vi "Read Waveform (Multiple).vi"(8 "error in (no error)":errorcluster, 9 "Maximum Time (5000 ms)":u32=5000, 10 "Channels":u16[](array[ring])=[1, 2] items=["Channel 1"=1, "Channel 2"=2], 11 "VISA resource name":refnum<visa-resource-name>) -> (0 "error out":errorcluster, 2 "Waveform Data":dbl[][](graph), 3 "VISA resource name out":refnum<visa-resource-name>)   [LabVIEW 2015, in "ZhiYuan ZDS Series for TCP.lvlib"]
doc: "Initiates an acquisition on all channels that you enabled with the Configure Channel VI. The VI waits for the acquisition to complete and returns the waveform for the <B>Source Channel</B> you specified. If the oscilloscope did not complete the acquisition within the time period you specify with the <B>Timeout</B> control, the VI returns a timeout error. A common cause for a timeout error is the acquisition was not triggered. For example, the trigger level is out of range of the waveform. \n\n<B>Note:</B> If your instrument does not support auto compensation for probe attenuation, you may need to adjust the scaling of the waveform data accordingly. This is handled automatically in the Configure Channel VI or can be done manually by multiplying the waveform data by the probe attenuation."
uses:
  ZhiYuan ZDS Series for TCP.lvlib
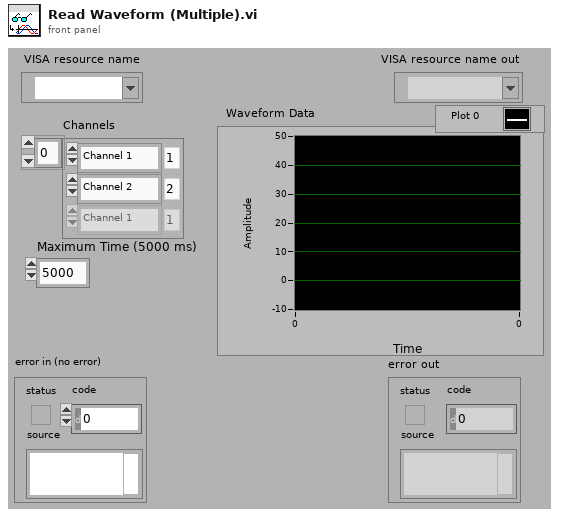
[diagram p1: front panel]
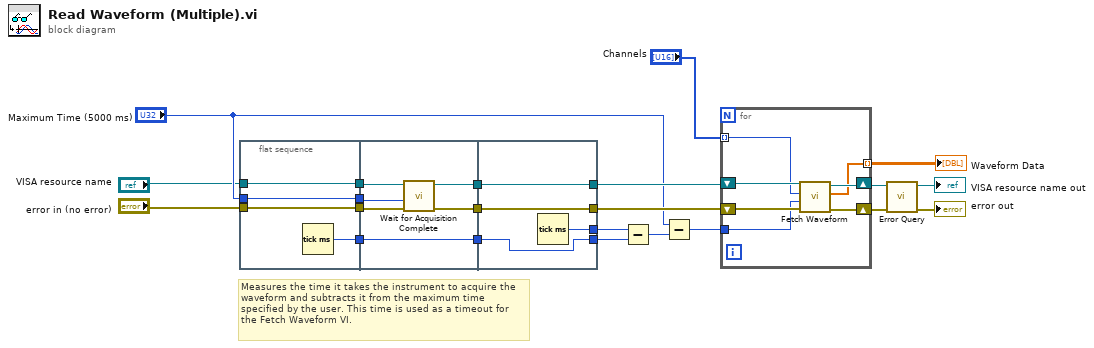
[diagram p0: block diagram]
diagram:
  # "Measures the time it takes the instrument to acquire the waveform and subtracts it from the maximum time specified by the user. This time is used as a timeout for the Fetch Waveform VI."
  n1 = flat-sequence {
    tunnel: "VISA resource name" -> [w25]
    tunnel: [w25] -> w9
    tunnel: "error in (no error)" -> [w24]
    tunnel: [w24] -> w8
    tunnel: "Maximum Time (5000 ms)" -> [w23]
    tunnel: [w23] -> w7
    tunnel: [w26] -> w6
    tunnel: w9 -> [w32]
    tunnel: [w31] -> w5
    tunnel: w8 -> [w30]
    tunnel: [w29] -> w4
    tunnel: w7 -> [w28]
    tunnel: w6 -> [w27]
    tunnel: [w27] -> w3
    tunnel: [w35] -> w13
    tunnel: w5 -> [w35]
    tunnel: [w34] -> w12
    tunnel: w4 -> [w34]
    tunnel: [w33] -> w15
    tunnel: w3 -> [w33]
    tunnel: [w36] -> w14
    frame #0 {
      n2 = Tick Count (ms)() -> (millisecond timer value=w26:u32)
    }
    frame #1 {
      n3 = call "Wait for Acquisition Complete.vi"("error in (no error)"=w30, "Maximum Time (10000 ms)"=w28, "VISA resource name"=w32) -> ("error out"=w29:errorcluster, "VISA resource name out"=w31:refnum<visa-resource-name>)  [unwired: 7 in]
    }
    frame #2 {
      n4 = Tick Count (ms)() -> (millisecond timer value=w36:u32)
    }
  }
  n5 = Subtract(x=w14, y=w15) -> (x-y=w16:u32)
  n6 = Subtract(x="Maximum Time (5000 ms)", y=w16) -> (x-y=w11:u32)
  n7 = for {
    shift-right: [w42] -> w19
    shift-left: w12 -> [w40]
    tunnel: "Channels" -> [w39] mode=indexing
    tunnel: [w38] -> w17 mode=indexing
    shift-right: [w43] -> w20
    shift-left: w13 -> [w41]
    tunnel: w11 -> [w37]
    n8 = call "Fetch Waveform.vi"("error in (no error)"=w40, "Timeout (5000 ms)"=w37, "Channel (1: Channel 1)"=w39, "VISA resource name"=w41) -> ("error out"=w42:errorcluster, "Waveform Data"=w38:dbl[], "VISA resource name out"=w43:refnum<visa-resource-name>)  [unwired: 5 in]
  }
  "Waveform Data" <- w17
  n9 = call "Error Query.vi"("error in (no error)"=w19, "VISA resource name"=w20) -> ("error out"=→"error out":errorcluster, "VISA resource name out"=→"VISA resource name out":refnum<visa-resource-name>)  [unwired: 6 in, 2 out]
